vi "PulseParseMW.vi"(1 "String":string) -> (0 "Full Pulse Array":T1(array[cluster]))   [LabVIEW 2017]
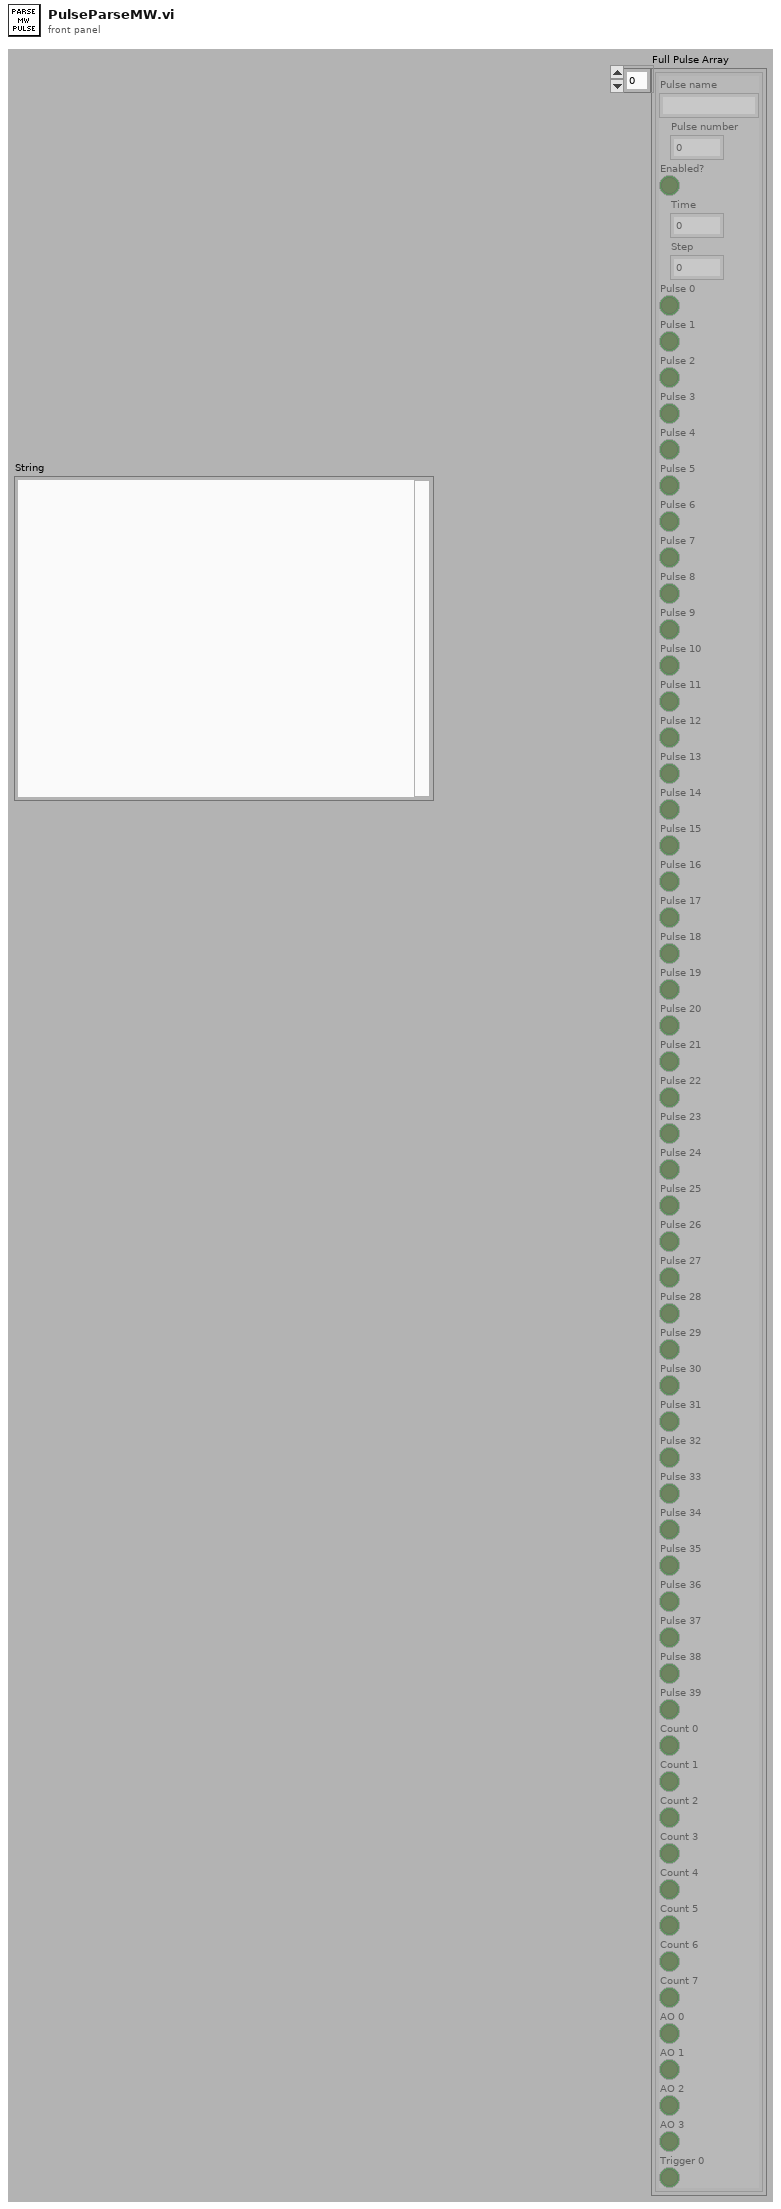
[diagram p1: front panel]
types:
  T1 = cluster{"Pulse name":string, "Pulse number":i32, "Enabled?":bool, "Time":dbl, "Step":dbl, "Pulse 0":bool, "Pulse 1":bool, "Pulse 2":bool, "Pulse 3":bool, "Pulse 4":bool, "Pulse 5":bool, "Pulse 6":bool, "Pulse 7":bool, "Pulse 8":bool, "Pulse 9":bool, "Pulse 10":bool, "Pulse 11":bool, "Pulse 12":bool, "Pulse 13":bool, "Pulse 14":bool, "Pulse 15":bool, "Pulse 16":bool, "Pulse 17":bool, "Pulse 18":bool, "Pulse 19":bool, "Pulse 20":bool, "Pulse 21":bool, "Pulse 22":bool, "Pulse 23":bool, "Pulse 24":bool, "Pulse 25":bool, "Pulse 26":bool, "Pulse 27":bool, "Pulse 28":bool, "Pulse 29":bool, "Pulse 30":bool, "Pulse 31":bool, "Pulse 32":bool, "Pulse 33":bool, "Pulse 34":bool, "Pulse 35":bool, "Pulse 36":bool, "Pulse 37":bool, "Pulse 38":bool, "Pulse 39":bool, "Count 0":bool, "Count 1":bool, "Count 2":bool, "Count 3":bool, "Count 4":bool, "Count 5":bool, "Count 6":bool, "Count 7":bool, "AO 0":bool, "AO 1":bool, "AO 2":bool, "AO 3":bool, "Trigger 0":bool}[]
  T2 = cluster{"Pulses":u64, "Time":dbl, "Step":dbl, "Enabled?":bool, "Pulse name":string, "Counts":u8, "Triggers":u8, "AOs":u8}
  T3 = cluster{"Pulse name":string, "Pulse number":i32, "Enabled?":bool, "Time":dbl, "Step":dbl, "Pulse 0":bool, "Pulse 1":bool, "Pulse 2":bool, "Pulse 3":bool, "Pulse 4":bool, "Pulse 5":bool, "Pulse 6":bool, "Pulse 7":bool, "Pulse 8":bool, "Pulse 9":bool, "Pulse 10":bool, "Pulse 11":bool, "Pulse 12":bool, "Pulse 13":bool, "Pulse 14":bool, "Pulse 15":bool, "Pulse 16":bool, "Pulse 17":bool, "Pulse 18":bool, "Pulse 19":bool, "Pulse 20":bool, "Pulse 21":bool, "Pulse 22":bool, "Pulse 23":bool, "Pulse 24":bool, "Pulse 25":bool, "Pulse 26":bool, "Pulse 27":bool, "Pulse 28":bool, "Pulse 29":bool, "Pulse 30":bool, "Pulse 31":bool, "Pulse 32":bool, "Pulse 33":bool, "Pulse 34":bool, "Pulse 35":bool, "Pulse 36":bool, "Pulse 37":bool, "Pulse 38":bool, "Pulse 39":bool, "Count 0":bool, "Count 1":bool, "Count 2":bool, "Count 3":bool, "Count 4":bool, "Count 5":bool, "Count 6":bool, "Count 7":bool, "AO 0":bool, "AO 1":bool, "AO 2":bool, "AO 3":bool, "Trigger 0":bool}
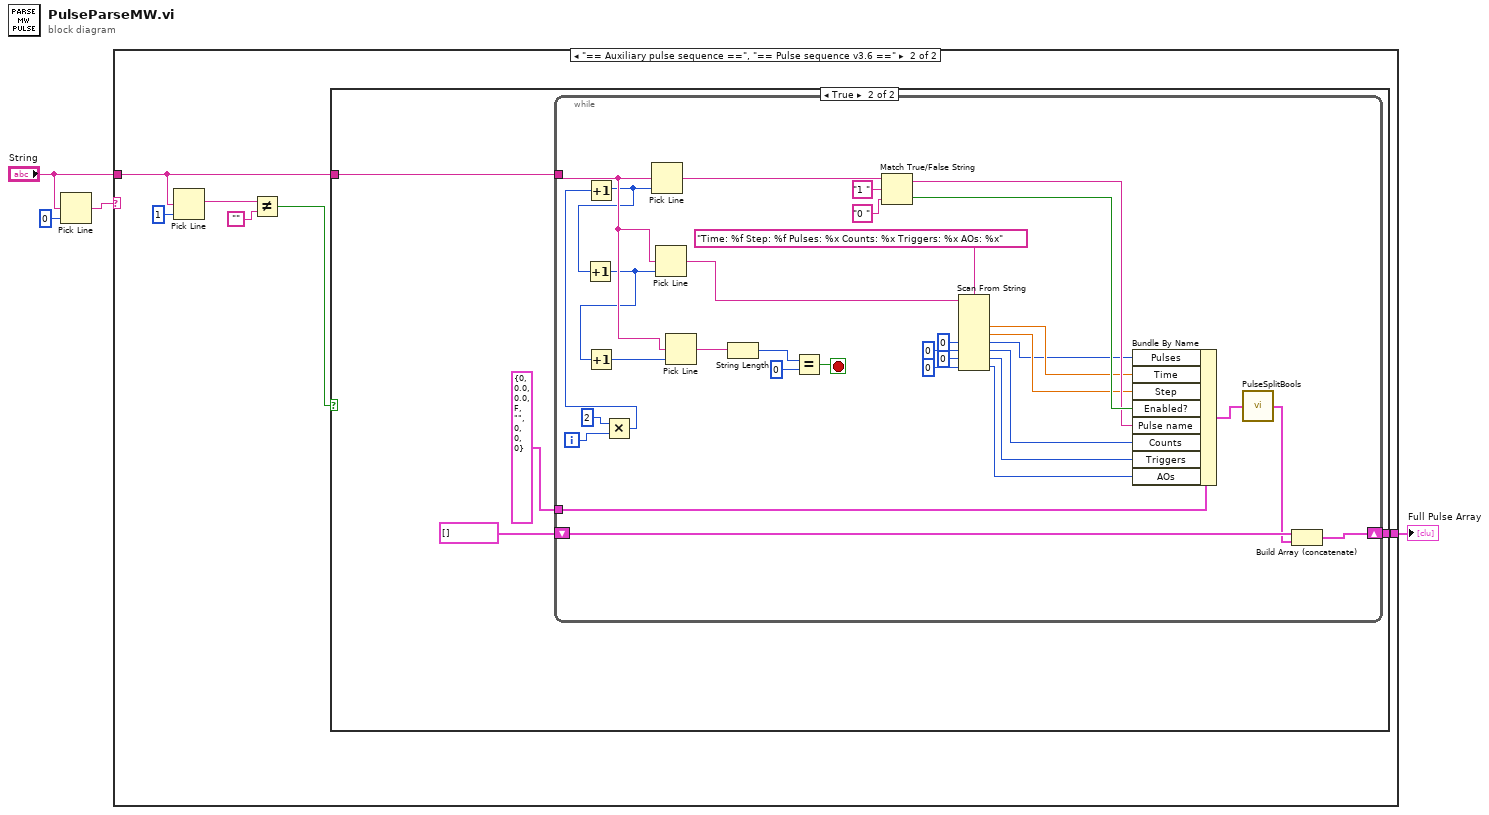
[diagram p0: block diagram]
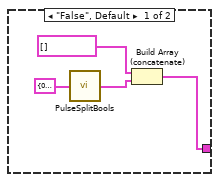
[diagram p2: hidden frame]
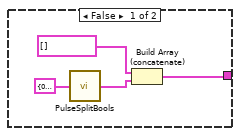
[diagram p3: hidden frame]
diagram:
  n1 = Pick Line(multi-line string="String", line index=0) -> (output string=w2:string)  [unwired: 1 in]
  n2 = case shown="\"== Auxiliary pulse sequence ==\", \"== Pulse sequence v3.6 ==\"" w2 {
    tunnel: [w7 w14] -> w1
    tunnel: "String" -> [_ w13]
    frame "False", Default {
      n3 = call "PulseSplitBools.vi"("Pulse input"=T2 {"Pulses"=0, "Time"=0.0, "Step"=0.0, "Enabled?"=FALSE, "Pulse name"="", "Counts"=0, "Triggers"=0, "AOs"=0} ("Combined pulse")) -> ("output cluster"=w5:T3)
      n4 = Build Array (concatenate)(T1 [] ("Full Pulse Array"), w5) -> (w7:T1)
    }
    frame "== Auxiliary pulse sequence ==", "== Pulse sequence v3.6 ==" {
      n5 = Pick Line(multi-line string=w13, line index=1) -> (output string=w10:string)  [unwired: 1 in]
      n6 = Not Equal?(x=w10, y="") -> (x != y?=w9:bool)
      n7 = case shown="True" w9 {
        tunnel: [w15 w21] -> w14
        tunnel: w13 -> [_ w19]
        frame False {
          n8 = call "PulseSplitBools.vi"("Pulse input"=T2 {"Pulses"=0, "Time"=0.0, "Step"=0.0, "Enabled?"=FALSE, "Pulse name"="", "Counts"=0, "Triggers"=0, "AOs"=0} ("Combined pulse")) -> ("output cluster"=w18:T3)
          n9 = Build Array (concatenate)(T1 [] ("Full Pulse Array"), w18) -> (w15:T1)
        }
        frame True {
          n10 = while {
            tunnel: w19 -> [w49]
            shift-right: [w42] -> w21
            shift-left: T1 [] ("Full Pulse Array") -> [w41]
            tunnel: T2 {"Pulses"=0, "Time"=0.0, "Step"=0.0, "Enabled?"=FALSE, "Pulse name"="", "Counts"=0, "Triggers"=0, "AOs"=0} ("Combined pulse") -> [w40]
            i -> [w48]
            stop <- w37 stop-if-true
            n11 = Multiply(x=2, y=w48) -> (x*y=w46:i32)
            n12 = Increment(x=w46) -> (x+1=w45:i32)
            n13 = Increment(x=w45) -> (x+1=w44:i32)
            n14 = Increment(x=w44) -> (x+1=w43:i32)
            n15 = Pick Line(multi-line string=w49, line index=w45) -> (output string=w53:string)  [unwired: 1 in]
            n16 = Pick Line(multi-line string=w49, line index=w44) -> (output string=w54:string)  [unwired: 1 in]
            n17 = Pick Line(multi-line string=w49, line index=w43) -> (output string=w50:string)  [unwired: 1 in]
            n18 = String Length(string=w50) -> (length=w39:i32)
            n19 = Equal?(x=w39, y=0) -> (x = y?=w37:bool)
            n20 = Match True/False String(2:"0 " ("false string"), 3:"1 " ("true string"), 4:w53) -> (0:w36:bool, 1:w35:string)
            n21 = Scan From String(format string="Time: %f Step: %f Pulses: %x Counts: %x Triggers: %x AOs: %x", input string=w54, default 3=u64 0 ("default value 3"), default 4=u8 0 ("default value 4"), default 5=u8 0 ("default value 5"), default 6=u8 0 ("default value 6")) -> (output 1=w33:dbl, output 2=w34:dbl, output 3=w29:u64, output 4=w25:u8, output 5=w24:u8, output 6=w23:u8)  [unwired: 4 in, 3 out]
            n22 = Bundle By Name(cluster=w40, "Pulses"=w29, "Time"=w33, "Step"=w34, "Enabled?"=w36, "Pulse name"=w35, "Counts"=w25, "Triggers"=w24, "AOs"=w23) -> (w32:T2)
            n23 = call "PulseSplitBools.vi"("Pulse input"=w32) -> ("output cluster"=w31:T3)
            n24 = Build Array (concatenate)(w41, w31) -> (w42:T1)
          }
        }
      }
    }
  }
  "Full Pulse Array" <- w1
